vi "delete action from sequence by index.vi"(8 "error in (no error)":errorcluster, 9 "index":i32, 10 "sequence name":string, 11 "Simple Sequencer TBM configuration in":refnum<class "Simple Sequencer TBM configuration.lvclass">) -> (0 "error out":errorcluster, 3 "Simple Sequencer TBM configuration out":refnum<class "Simple Sequencer TBM configuration.lvclass">)   [LabVIEW 2014, in "Simple Sequencer TBM configuration.lvclass"]
doc: "Deletes the action found at index in the specified sequence."
uses:
  Simple Sequencer TBM configuration.lvclass
  Simple Sequencer TBM configuration.lvclass/Simple Sequencer TBM configuration.ctl
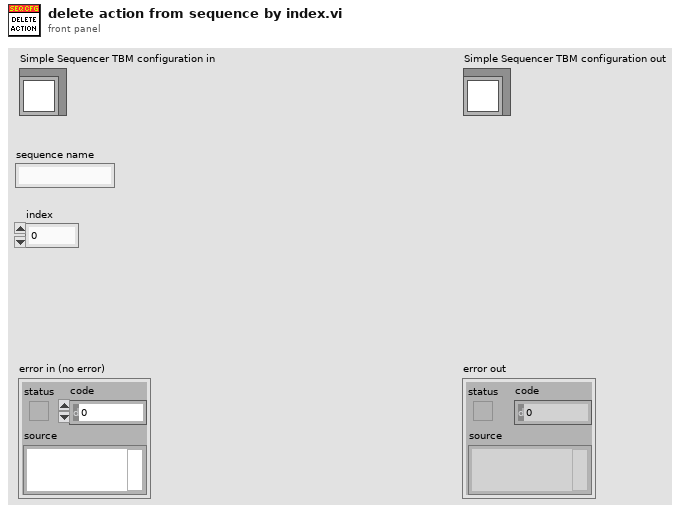
[diagram p1: front panel]
types:
  T1 = typedef "Simple Sequencer TBM configuration.lvclass/sequence definition.ctl" = cluster{"sequence name":string, "action configs":refnum<class "action configuration.lvclass">[]}
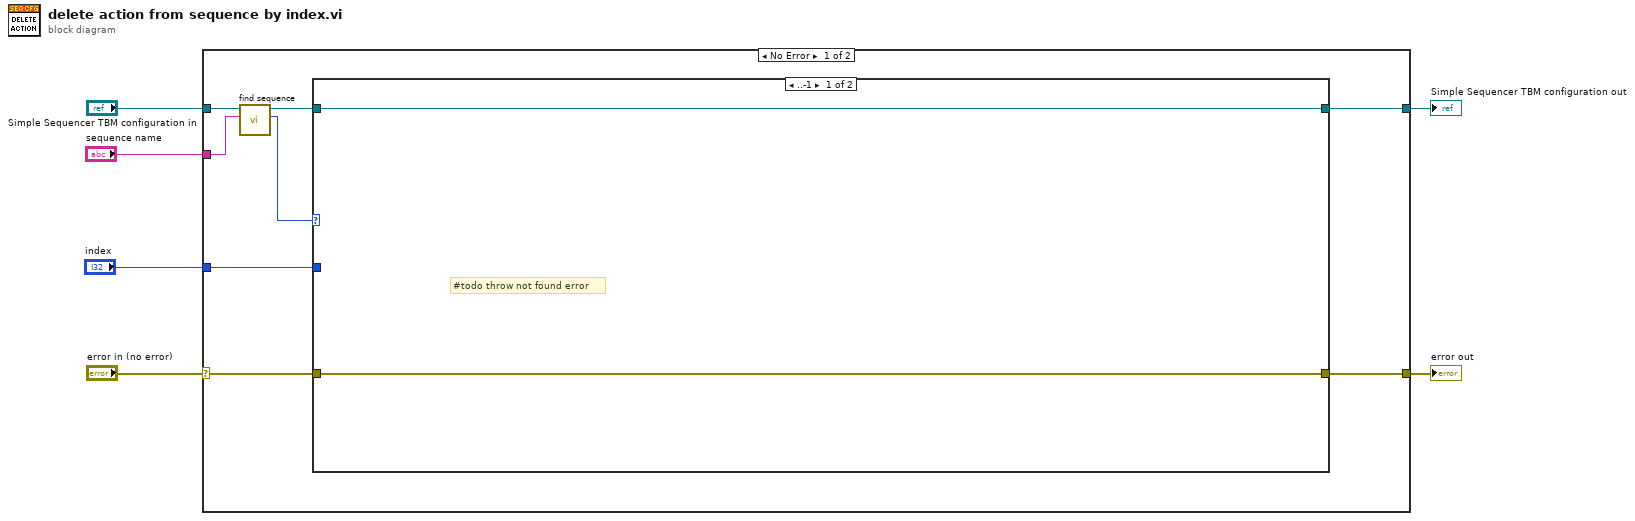
[diagram p0: block diagram]
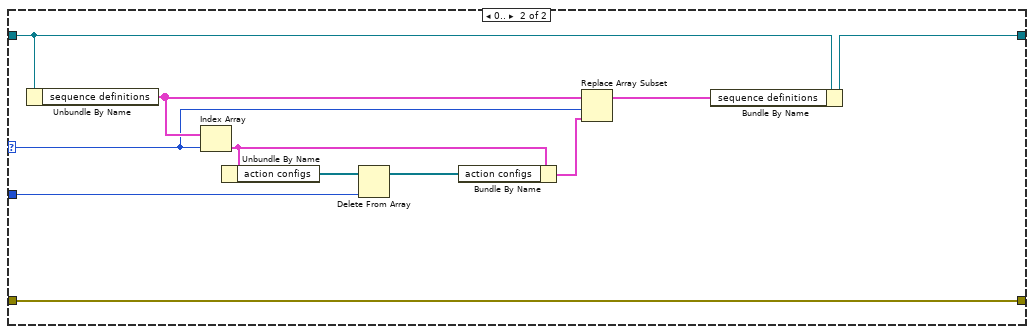
[diagram p2: hidden frame]
diagram:
  n1 = case shown="No Error" "error in (no error)" {
    selector: "error in (no error)" -> [w10 w29]
    tunnel: [w9 w29] -> w5
    tunnel: [w7 w28] -> w3
    tunnel: "Simple Sequencer TBM configuration in" -> [w14 w28]
    tunnel: "sequence name" -> [w12 _]
    tunnel: "index" -> [w8 _]
    frame No Error {
      n2 = call "find sequence.vi"("sequence name"=w12, "Simple Sequencer TBM configuration in"=w14) -> ("index"=w11:i32, "Simple Sequencer TBM configuration out"=w13:refnum<class "Simple Sequencer TBM configuration.lvclass">)  [unwired: 8 in]
      n3 = case shown="..-1" w11 {
        selector: w11 -> [_ w22]
        tunnel: w13 -> [w15 w20]
        tunnel: w10 -> [w16 w17]
        tunnel: [w16 w17] -> w9
        tunnel: w8 -> [_ w26]
        tunnel: [w15 w18] -> w7
        frame ..-1 {
          # "#todo throw not found error"
        }
        frame 0.. {
          n4 = Unbundle By Name(w20) -> ("sequence definitions"=w23:T1[])
          n5 = Index Array(array=w23, index=w22) -> (element=w25:T1)
          n6 = Unbundle By Name(w25) -> ("action configs"=w27:refnum<class "action configuration.lvclass">[])
          n7 = Delete From Array(array=w27, index=w26) -> (array with subset deleted=w24:refnum<class "action configuration.lvclass">[])  [unwired: 1 in, 1 out]
          n8 = Bundle By Name(cluster=w25, "action configs"=w24) -> (w21:T1)
          n9 = Replace Array Subset(array=w23, new element=w21, index=w22) -> (w19:T1[])
          n10 = Bundle By Name(cluster=w20, "sequence definitions"=w19) -> (w18:refnum<class "Simple Sequencer TBM configuration.lvclass">)
        }
      }
    }
    frame Error {
    }
  }
  "error out" <- w5
  "Simple Sequencer TBM configuration out" <- w3
